vi "SVT Spectrum Peak Search (N Ch).vi"(0 "spectra":cluster{"x0":dbl, "dx":dbl, "magnitude":dbl[]}[](array[cluster]) {"magnitude" format="%.2f"; "dx" format="%.2f"; "x0" format="%.2f"}, 1 "peak search settings":T6={"single/multiple"=enum."Multiple Peaks", "threshold"=inf} {"threshold" format="%.2f"}, 4 "spectrum info":T1[](array[typedef]) {"x-axis units" items=["time"=0, "frequency"=1, "quefrency"=2, "revolutions"=3, "order"=4, "rpm"=11, "rad/s"=21, "index"=65535]; "weighting filter" items=["Linear", "A-weighting", "B-weighting", "C-weighting", "ITU-R 468-4", "Dolby", "CCITT", "C-message"]; "dB reference [EU]" format="%.2f"; "engineering units" items=["custom..."=0, "V"=1, "A"=21, "Pa"=2, "N"=20, "g"=3, "m/s^2"=4, "m/s"=5, "m"=6, "mm/s"=12, "mm"=13, "microns/s"=14, "microns"=15, "in/s^2"=7, "in/s"=8, "in"=9, "mils/s"=10, "mils"=11, "rad/s^2"=16, "rad/s"=17, "rad"=18, "strain"=19]; "spectral info"."window" items=["None "=0, "Hanning"=1, "Hamming"=2, "Blackman-Harris"=3, "Exact Blackman"=4, "Blackman"=5, "Flat Top"=6, "4 Term B-Harris "=7, "7 Term B-Harris"=8, "Low Sidelobe"=9, "Force - Exponential"=10, "Gaussian"=62]}, 5 "error in (no error)":errorcluster) -> (14 "peaks":cluster{"freq. or order":dbl, "value":dbl}[][](array[cluster]) {"value" format="%.2f"; "freq. or order" format="%.2f"}, 15 "number of peaks":i32[](array[numeric]), 16 "unit labels":string[](array[string]), 19 "error out":errorcluster)   [LabVIEW 2017]
doc: "Performs a peak search on a spectrum or spectra. The spectrum or spectra can be in either the frequency domain or the order domain. Detects single or multiple peaks in Power, PSD, and COP spectra. You can use this polymorphic VI to analyze a single spectrum or N spectra. The data type you wire to the <B>spectrum</B> input determines the polymorphic instance to use."
uses:
  <vilib>/addons/Sound and Vibration/compatibility/Controls/svl_Spectrum Info (enhanced).ctl
  <vilib>/addons/Sound and Vibration/compatibility/Controls/svl_Spectrum Type.ctl
  <vilib>/addons/Sound and Vibration/compatibility/Controls/svl_Engineering Units Text Ring.ctl
  <vilib>/addons/Sound and Vibration/compatibility/Controls/svl_Weighting Filter Text Ring.ctl
  <vilib>/addons/Sound and Vibration/compatibility/Controls/svl_Complimentary Spectrum Units.ctl
  <vilib>/addons/_NISVFA/_Spectrum Processing/subVIs/svfa_Spectrum Peak Search.vi
  <vilib>/addons/_NISVFA/_Shared subVIs/Common/svc_Spectrum Units.vi
  <vilib>/addons/_NISVFA/_Spectrum Processing/subVIs/svfa_Peak Rough Search Indices.vi
  <vilib>/addons/_NISVFA/_Shared subVIs/Common/svc_Get Weighting Enum and Labels.vi
  <vilib>/addons/_NISVFA/_Shared subVIs/Common/svc_Unit Label Lexical Class.vi
  <vilib>/addons/_NISVFA/_Shared subVIs/Common/svc_Engineering Units to Unit Label.vi
  <vilib>/addons/_NISVFA/_Shared subVIs/Common/svc_Format Value (DBL).vi
  <vilib>/addons/_NISVFA/_Spectrum Processing/subVIs/svfa_Three Finger Peak Search.vi
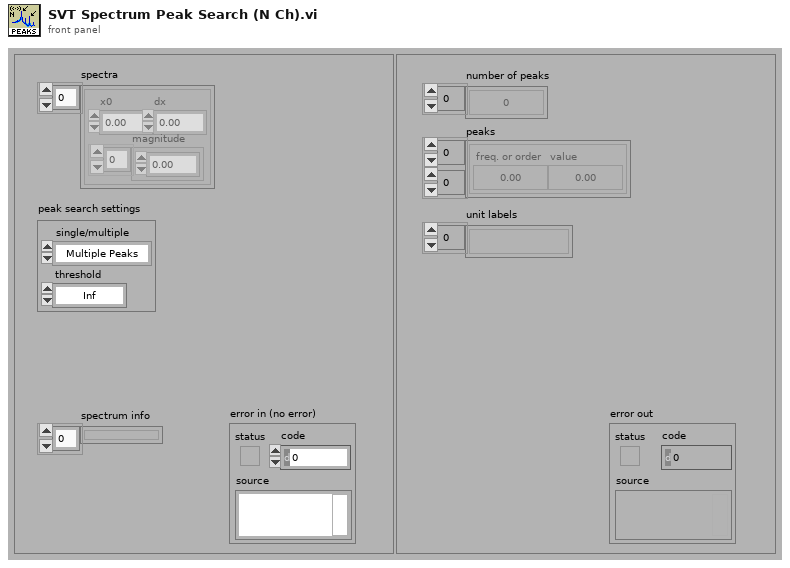
[diagram p1: front panel]
types:
  T1 = typedef "svl_Spectrum Info (enhanced).ctl" = cluster{"channel name":string, "description":string, "x-axis units":u16, "spectral info":cluster{"spectrum type":T2, "linear/dB":enum16{"linear", "dB"}, "window":u16, "window size":i32, "FFT size":i32}, "engineering units":T3, "custom label":string, "dB reference [EU]":dbl, "peak units":enum16{"rms", "peak", "peak-peak"}, "weighting filter":T4, "spectral density?":bool, "unit label":string, "spectrum skewed?":bool, "complimentary spectrum units":T5}
  T2 = typedef "svl_Spectrum Type.ctl" = enum16{"FFT Spectrum [complex]", "Amplitude [Magnitude]", "Power [Magnitude^2]", "Cross Spectrum [complex]", "Frequency Response [Complex]"}
  T3 = typedef "svl_Engineering Units Text Ring.ctl" = u16
  T4 = typedef "svl_Weighting Filter Text Ring.ctl" = u16
  T5 = typedef "svl_Complimentary Spectrum Units.ctl" = enum16{"none", "radians", "degrees", "cycles", "imaginary"}
  T6 = cluster{"single/multiple":enum16{"Multiple Peaks", "Single Max Peak"}, "threshold":dbl}
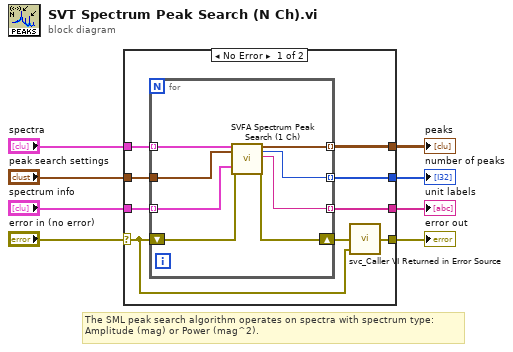
[diagram p0: block diagram]
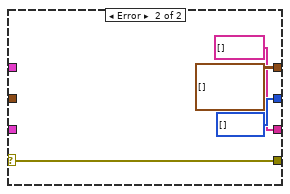
[diagram p2: hidden frame]
diagram:
  # "The SML peak search algorithm operates on spectra with spectrum type:\nAmplitude (mag) or Power (mag^2)."
  n1 = case shown="No Error" "error in (no error)" {
    selector: "error in (no error)" -> [w9 w29]
    tunnel: "peak search settings" -> [w17 _]
    tunnel: [w16 cluster{"frequency":dbl, "value":dbl}[][] [] ("peaks")] -> w7
    tunnel: [w15 i32[] []] -> w6
    tunnel: "spectrum info" -> [w14 _]
    tunnel: [w10 w29] -> w4
    tunnel: "spectra" -> [w12 _]
    tunnel: [w11 string[] []] -> w2
    frame No Error {
      n2 = for {
        tunnel: w12 -> [w25] mode=indexing
        tunnel: w17 -> [w20]
        tunnel: [w24] -> w16 mode=indexing
        tunnel: w14 -> [w21] mode=indexing
        tunnel: [w23] -> w15 mode=indexing
        shift-right: [w18] -> w13
        shift-left: w9 -> [w19]
        tunnel: [w22] -> w11 mode=indexing
        n3 = call <vilib>:"SVFA Spectrum Peak Search (1 Ch).vi"("spectrum"=w25, "peak search settings"=w20, "spectrum info in"=w21, "error in (no error)"=w19) -> ("peaks"=w24:cluster{"freq. or order":dbl, "value":dbl}[], "number of peaks"=w23:i32, "unit label"=w22:string, "error out"=w18:errorcluster)  [unwired: 11 in, 1 out]
      }
      n4 = call <vilib>:"svc_Caller VI Returned in Error Source.vi"("warning input to caller"=w9, "error in (no error)"=w13) -> ("error out"=w10:errorcluster)  [unwired: 3 in]
    }
    frame Error {
    }
  }
  "error out" <- w4
  "number of peaks" <- w6
  "peaks" <- w7
  "unit labels" <- w2
